vi "Patel_4th_Gettingstarted_12-1-16.vi"   [LabVIEW 2014, in "Patel_4th_RoboTest_11-10-16.lvrbt"]
uses:
  Patel_4th_RoboTest_11-10-16.lvrbt
  <vilib>/NXT/Block Support/NXT_OutputPort.ctl
  <vilib>/NXT/NXTIO Xnodes/NXTIONodeSubVIs/NXTMoveMotors.vi
  <vilib>/NXT/Dual Mode Library/Waits/Wait_Num.vi
  <vilib>/NXT/Subs/LVHSConnector.ctl
  <vilib>/NXT/NXTIO Xnodes/AddressXNode/NXTIOAddress.xnode
  <vilib>/NXT/NXTIO Xnodes/NXTIOXNode/NXTIO.xnode
  <vilib>/NXT/LegoClasses/BrickReference/BrickReference.lvclass
types:
  T1 = typedef "NXT_OutputPort.ctl" = u8
  T2 = typedef "LVHSConnector.ctl" = refnum<class "BrickReference.lvclass">
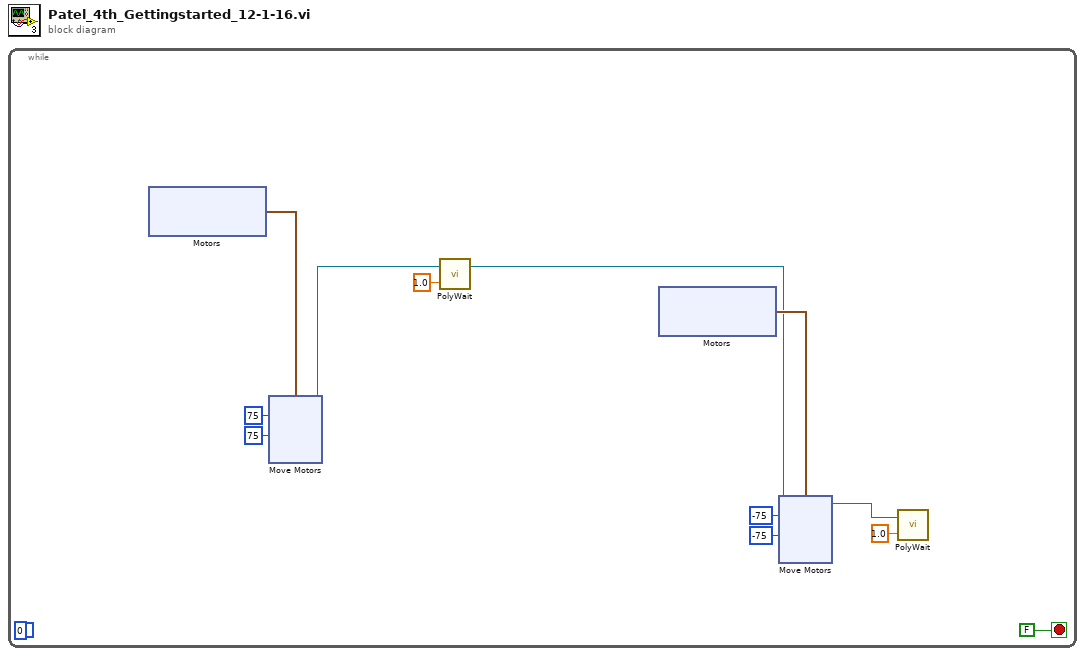
[diagram p0: block diagram]
diagram:
  n1 = while {
    stop <- FALSE stop-if-true
    (unwired) 0
    n2 = xnode "Motors"() -> ("Motor"=w12:cluster{"Port":T1, "Port":T1})
    n3 = xnode "Move Motors"("Power/Speed 2"=i8 75, "Power/Speed 1"=i8 75, "Motors"=w12) -> ("NXT/EV3"=w8:T2)  [unwired: 1 in]
    n4 = call-poly <vilib>:"PolyWait.vi"("Time (1 sec)"=sgl 1.0, "NXT/EV3"=w8) -> ("NXT/EV3"=w4:T2)  [unwired: 2 in]
    n5 = xnode "Motors"() -> ("Motor"=w7:cluster{"Port":T1, "Port":T1})
    n6 = xnode "Move Motors"("Power/Speed 2"=i8 -75, "Power/Speed 1"=i8 -75, "Motors"=w7, "NXT/EV3"=w4) -> ("NXT/EV3"=w3:T2)
    n7 = call-poly <vilib>:"PolyWait.vi"("Time (1 sec)"=sgl 1.0, "NXT/EV3"=w3) -> ()  [unwired: 2 in, 1 out]
  }
